vi "Add New Transactions.vi"(8 "error in (no error)":errorcluster, 10 "Importing Transactions":refnum<class "Statement.lvclass">, 11 "Database in":refnum<class "Database.lvclass">) -> (0 "error out":errorcluster, 1 "Num Recs to Insert":i32, 3 "Database out":refnum<class "Database.lvclass">)   [LabVIEW 2018, in "Database.lvclass"]
uses:
  Database.lvclass
  Statement/Statement.lvclass
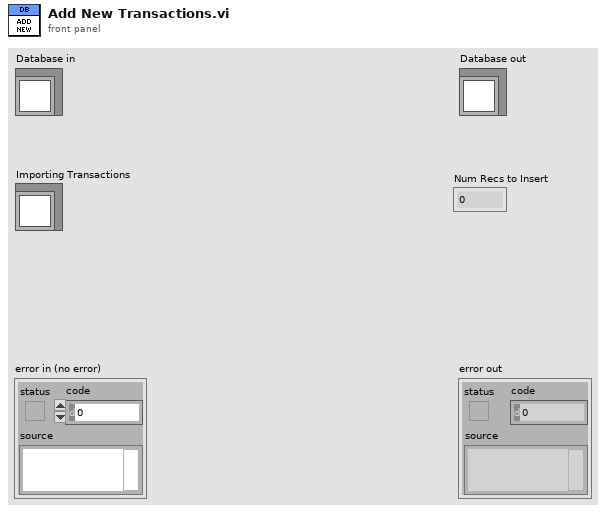
[diagram p1: front panel]
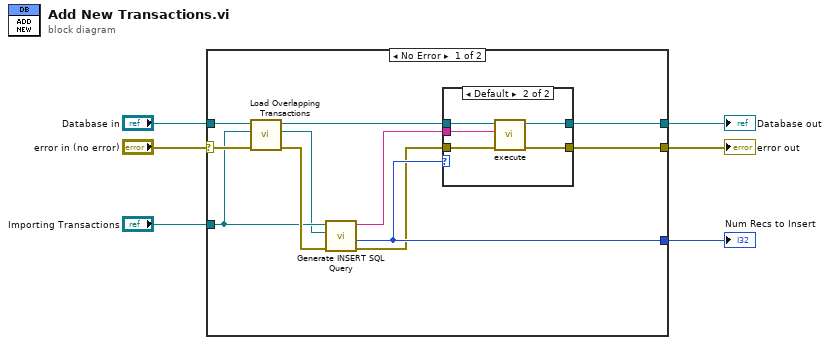
[diagram p0: block diagram]
diagram:
  n1 = case shown="No Error" "error in (no error)" {
    selector: "error in (no error)" -> [w9 w25]
    tunnel: [w16 _] -> w6
    tunnel: "Database in" -> [w12 w26]
    tunnel: [w14 w26] -> w4
    tunnel: [w13 w25] -> w3
    tunnel: "Importing Transactions" -> [w8 _]
    frame No Error {
      n2 = call "Load Overlapping Transactions.vi"("error in (no error)"=w9, "Proposed Transactions"=w8, "Database in"=w12) -> ("error out"=w10:errorcluster, "Existing Transactions"=w7:refnum<class "Statement.lvclass">, "Database out"=w11:refnum<class "Database.lvclass">)  [unwired: 6 in]
      n3 = call-dynamic "Generate INSERT SQL Query.vi"("error in (no error)"=w10, "Overlappping Records"=w7, "Importing Transactions"=w8) -> ("error out"=w15:errorcluster, "Num Recs to Insert"=w16:i32, "INSERT Query"=w17:string)  [unwired: 6 in]
      n4 = case shown="Default" w16 {
        tunnel: w11 -> [w19 w24]
        tunnel: [w19 w23] -> w14
        tunnel: w15 -> [w18 w22]
        tunnel: [w18 w20] -> w13
        tunnel: w17 -> [_ w21]
        frame 0 {
        }
        frame Default {
          n5 = call "execute.vi"("error in (no error)"=w22, "SQL query"=w21, "Database in"=w24) -> ("error out"=w20:errorcluster, "Database out"=w23:refnum<class "Database.lvclass">)  [unwired: 7 in]
        }
      }
    }
    frame Error {
    }
  }
  "error out" <- w3
  "Database out" <- w4
  "Num Recs to Insert" <- w6
